vi "Stop Task.vi"(8 "error in (no error)":errorcluster, 11 "DAQmx Actor in":refnum<class "DAQmx Actor.lvclass">) -> (0 "error out":errorcluster, 3 "DAQmx Actor out":refnum<class "DAQmx Actor.lvclass">)   [LabVIEW 2024, in "DAQmx Actor.lvlib" / "DAQmx Actor.lvclass"]
uses:
  DAQmx Actor.lvclass
  DAQmx Actor.lvclass/DAQmx Actor.ctl
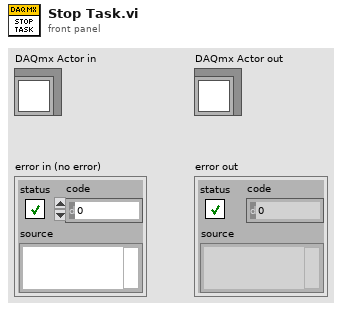
[diagram p1: front panel]
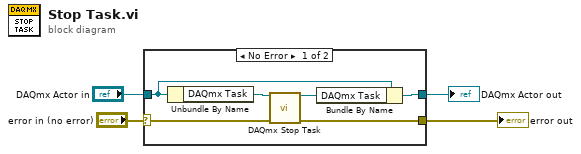
[diagram p0: block diagram]
diagram:
  n1 = case shown="No Error" "error in (no error)" {
    selector: "error in (no error)" -> [w9 w12]
    tunnel: [w8 w12] -> w3
    tunnel: [w5 w11] -> w1
    tunnel: "DAQmx Actor in" -> [w7 w11]
    frame No Error {
      n2 = Unbundle By Name(w7) -> ("DAQmx Task"=w10:refnum<k21>)
      n3 = call <vilib>:"DAQmx Stop Task.vi"("task/channels in"=w10, "error in"=w9) -> ("task out"=w6:refnum<k21>, "error out"=w8:errorcluster)  [unwired: 12 in]
      n4 = Bundle By Name(cluster=w7, "DAQmx Task"=w6) -> (w5:refnum<class "DAQmx Actor.lvclass">)
    }
    frame Error {
    }
  }
  "error out" <- w3
  "DAQmx Actor out" <- w1
